vi "Tegam4040 -- GetCalibrationMode.vi"(8 "error in (no error)":errorcluster, 11 "Instrument Session Handle In":u32 format="%x") -> (0 "error out":errorcluster, 2 "Calibration":T1(ring), 3 "Instrument Session Handle Out (dupl)":u32 format="%x")   [LabVIEW 2010]
panel:
  out "VISA Error Code":i32 format="%x"
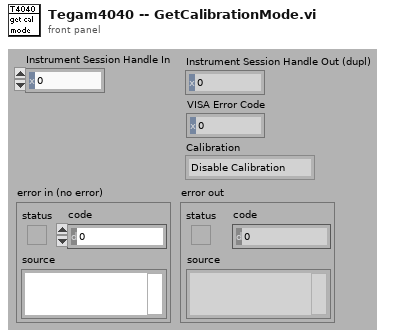
[diagram p1: front panel]
types:
  T1 = enum16{"Disable Calibration", "Enable Calibration"}
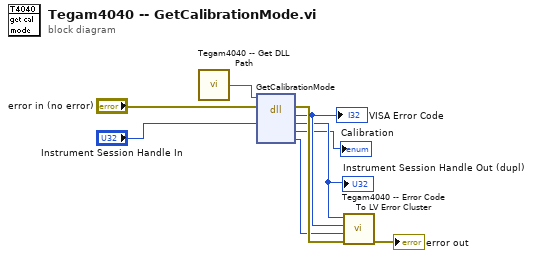
[diagram p0: block diagram]
diagram:
  n1 = call "Tegam4040 -- Get DLL Path.vi"() -> ("DLL Path"=w6:path)  [unwired: 8 in]
  n2 = dll-call lib="C:/Documents and Settings/Administrator/My Documents/Visual Studio 2005/Projects/Tegam4040CDriver/debug/Tegam4040CDriver.dll" fn="GetCalibrationMode" ("Tegam4040CDriver.dll:Close4040")(path in=w6, error in="error in (no error)", "instrSession"="Instrument Session Handle In") -> (error out=w8:errorcluster, "status"=w4:i32, "instrSession"=w3:u32, "calibrationMode"=→"Calibration":u16, "driverError"=w1:i32)  [unwired: 3 in, 1 out]
  "VISA Error Code" <- w4
  "Instrument Session Handle Out (dupl)" <- w3
  n3 = call "Tegam4040 -- Error Code To LV Error Cluster.vi"("error in (no error)"=w8, "Driver Error Code"=w1, "VISA Error Code"=w4, "Instrument Session Handle"=w3) -> ("error out"=→"error out":errorcluster)  [unwired: 7 in]
